vi "TestDCMotors.vi"() -> ()   [LabVIEW 2020]
uses:
  <vilib>/Platform/TimedLoop/XDataNode/timing_clust.ctl
  <vilib>/Platform/TimedLoop/XDataNode/nitl_modes.ctl
  <vilib>/Platform/TimedLoop/XDataNode/wakeup.ctl
  <vilib>/High Genius/HG_WSI_Tookit/Dependencies/Library/CAN/CAN.lvclass
  C:/Program Files (x86)/National Instruments/LabVIEW 2020/vi.lib/High Genius/HG_WSI_Tookit/Dependencies/Library/HG_LIB/HG_LIB.lvclass
  <vilib>/High Genius/HG_WSI_Tookit/Dependencies/Library/Digital Input and Output/Digital Input and Output.lvclass
  <vilib>/High Genius/HG_WSI_Tookit/Dependencies/Library/PWM/PWM.lvclass
  <vilib>/High Genius/HG_WSI_Tookit/Dependencies/Library/TitanENC/TitanENC.lvclass
  <vilib>/Platform/TimedLoop/XDataNode/XDataNode.xnode
  <vilib>/Platform/TimedLoop/XDataNode/XDNodeRunTimeDep.lvlib
  <vilib>/High Genius/HG_WSI_Tookit/Dependencies/Library/HG_LIB/HG_LIB.lvclass
panel:
  in  "s":bool
  in  "error in (no error)":errorcluster
  in  "Servo 1":T1={"Servo 1"=25.6734693877551, "Servo 2"=20.836734693877553, "Servo 3"=0.0} {"Servo 3" min=0.0 max=255.0 step=1.0 scale=10.0..40.0; "Servo 2" min=0.0 max=255.0 step=1.0 scale=10.0..40.0; "Servo 1" min=0.0 max=255.0 step=1.0 scale=10.0..40.0}
  out "Limit L":bool
  out "Limit H":bool
  in  "Motors Renum":cluster{"Num":i32, "Directly":bool, "KM":dbl}[](array[cluster])=[{"Num"=1, "Directly"=TRUE, "KM"=1.0}, {"Num"=3, "Directly"=FALSE, "KM"=1.0}, {"Num"=0, "Directly"=FALSE, "KM"=1.0}, {"Num"=2, "Directly"=TRUE, "KM"=1.0}]
  out "output cluster":T2
  out "Z":dbl
  out "Distance":cluster{"X":dbl, "Y":dbl}
  in  "Reset YAW":bool
  out "YAW (degree)":dbl
  in  "Start":bool
  in  "Drive On":bool
  in  "Drive":dbl[](array[slide])=[0.0, 0.0, -0.01, 1.0] step=1.0 scale=-100.0..100.0
  out "Waveform Chart":i32(graph)
  out "ENC/dt":T3
  out "RPM":T4
  out "ENC True":T5
  out "ENC":T5
  in  "Input":dbl[](array[slide])=[0.0, 0.0, -0.01, 1.0] step=1.0 scale=-100.0..100.0
  in  "Reset Enc":bool
  out "error out":errorcluster
  in  "stop":bool
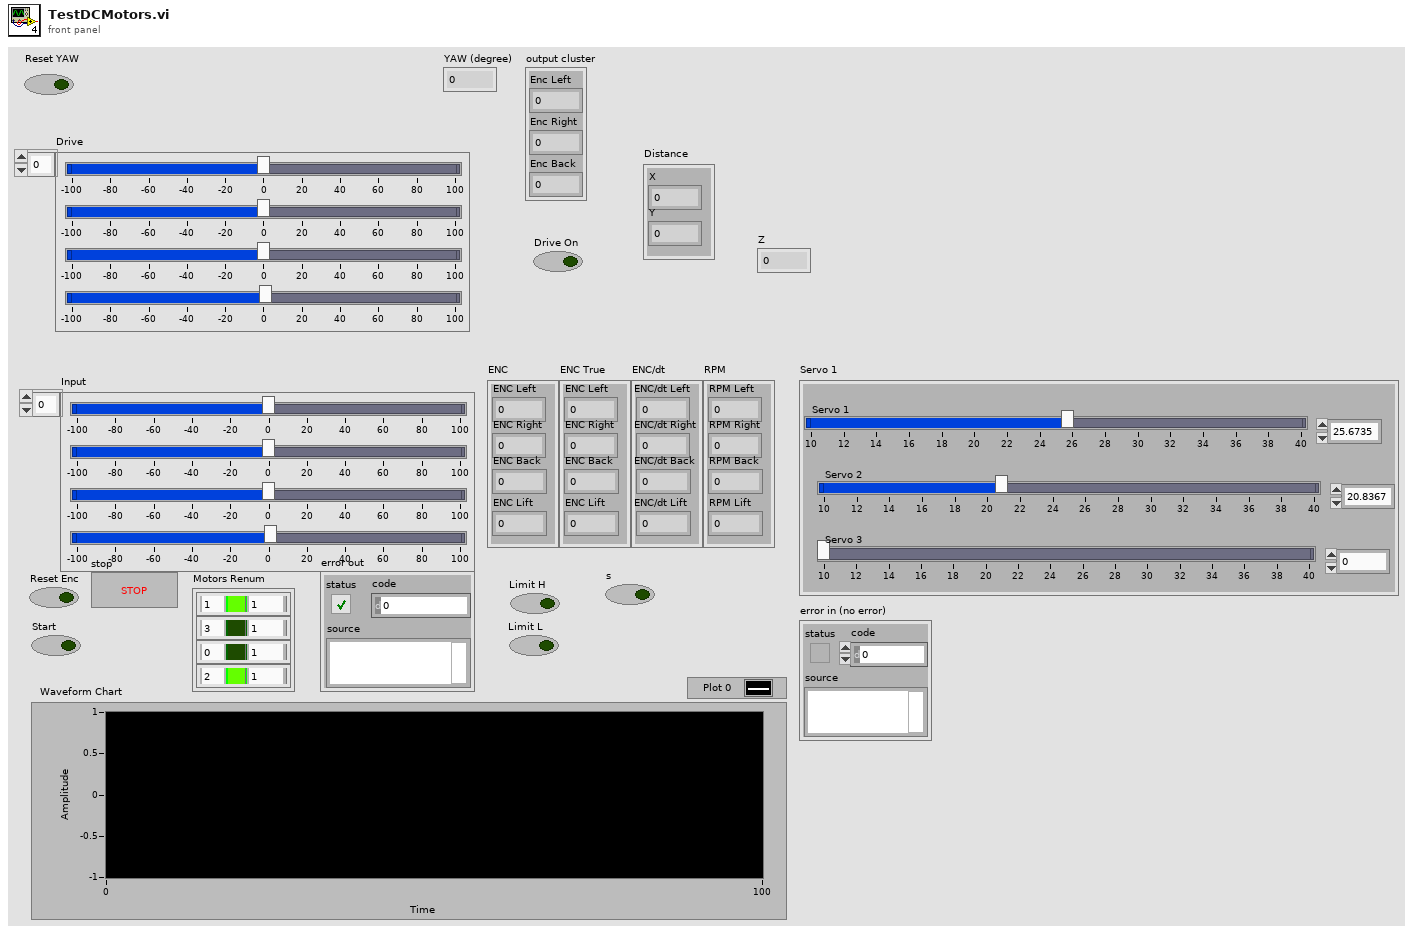
[diagram p1: front panel]
types:
  T1 = cluster{"Servo 1":dbl, "Servo 2":dbl, "Servo 3":dbl}
  T2 = cluster{"Enc Left":dbl, "Enc Right":dbl, "Enc Back":dbl}
  T3 = cluster{"ENC/dt Left":i32, "ENC/dt Right":i32, "ENC/dt Back":i32, "ENC/dt Lift":i32}
  T4 = cluster{"RPM Left":i32, "RPM Right":i32, "RPM Back":i32, "RPM Lift":i32}
  T5 = cluster{"ENC Left":i32, "ENC Right":i32, "ENC Back":i32, "ENC Lift":i32}
  T6 = cluster{"TitanENC 0":refnum<class "TitanENC.lvclass">, "TitanENC 1":refnum<class "TitanENC.lvclass">, "TitanENC 2":refnum<class "TitanENC.lvclass">, "TitanENC 3":refnum<class "TitanENC.lvclass">}
  T7 = cluster{"Limit H":refnum<class "Digital Input and Output.lvclass">, "Limit L":refnum<class "Digital Input and Output.lvclass">}
  T8 = cluster{"Servo 1":refnum<class "PWM.lvclass">, "Servo 2":refnum<class "PWM.lvclass">, "Servo 3":refnum<class "PWM.lvclass">}
  T9 = typedef "XDNodeRunTimeDep.lvlib/timing_clust.ctl" = cluster{"Expected End [f-1]":u64, "Actual End [f-1]":u64, "Finished Late? [f-1]":bool, "Expected End [i-1]":u64, "Actual End [i-1]":u64, "Finished Late? [i-1]":bool, "Expected Start [i]":u64, "Actual Start [i]":u64, "Expected Start [f]":u64, "Actual Start [f]":u64, "Source Name":string, "Structure Name":string, "Period":i64, "Deadline":i64, "Offset":i64, "Start":i64, "Priority":i32, "Timeout":i32, "Mode":T10, "Wakeup Reason":T11, "Error":errorcluster, "Source Type":string, "Secondary Source Type":string, "Global End Time":u64, "Global Start Time":u64, "Frame Duration":u64, "Iteration Duration":u64, "Assigned CPU":i32, "I/O Scan Engine Mode":u32}
  T10 = typedef "XDNodeRunTimeDep.lvlib/nitl_modes.ctl" = enum32{"No Change", "Process missed periods, maintain original phase", "Discard missed periods, maintain original phase", "Process missed periods, ignore original phase", "Discard missed periods, ignore original phase"}
  T11 = typedef "XDNodeRunTimeDep.lvlib/wakeup.ctl" = enum32{"Normal", "Aborted", "Asynchronous wakeup", "Timing source error", "Timed loop error", "Timeout"}
  T12 = cluster{"Limit H out":refnum<class "Digital Input and Output.lvclass">, "Limit L out":refnum<class "Digital Input and Output.lvclass">}
  T13 = cluster{"Servo 1 out":refnum<class "PWM.lvclass">, "Servo 2 out":refnum<class "PWM.lvclass">, "Servo 3 out":refnum<class "PWM.lvclass">}
  T14 = cluster{"TitanENC out":refnum<class "TitanENC.lvclass">, "TitanENC out":refnum<class "TitanENC.lvclass">, "TitanENC out":refnum<class "TitanENC.lvclass">, "TitanENC out":refnum<class "TitanENC.lvclass">}
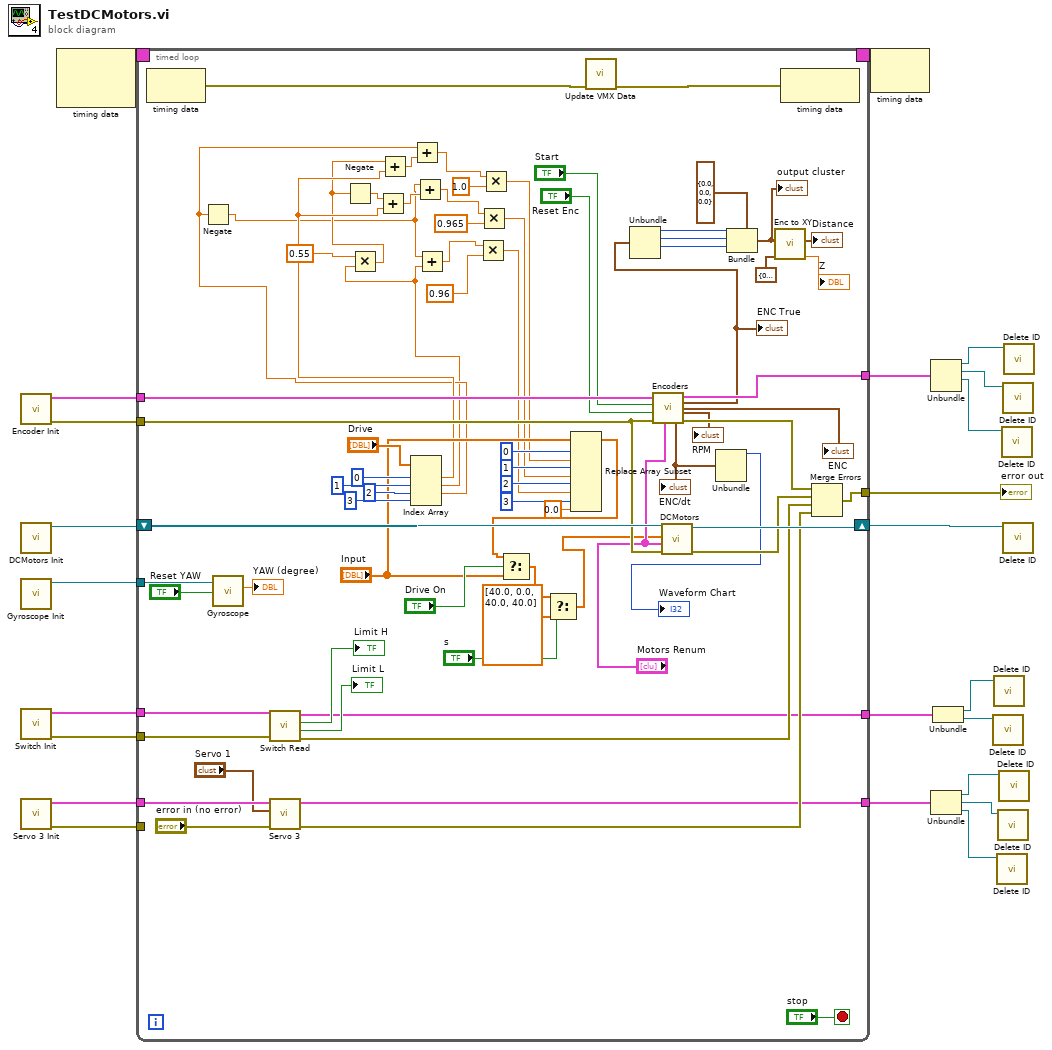
[diagram p0: block diagram]
diagram:
  n1 = call "Encoder Init.vi"() -> ("error out"=w14:errorcluster, "TitanENC out"=w15:T6)  [unwired: 10 in]
  n2 = call "DCMotors Init.vi"() -> ("DC Motors"=w13:refnum<class "CAN.lvclass">)  [unwired: 10 in, 1 out]
  n3 = call "Gyroscope Init.vi"() -> ("Gyroscope"=w12:refnum<class "IMU.lvclass">)  [unwired: 10 in, 1 out]
  n4 = call "Switch Init.vi"() -> ("error out"=w10:errorcluster, "Switch"=w11:T7)  [unwired: 10 in]
  n5 = call "Servo 3 Init.vi"() -> ("error out"=w8:errorcluster, "Servo"=w9:T8)  [unwired: 10 in]
  n6 = node-c288() -> (w23:T9)  [unwired: 2 in]
  n7 = timed-loop {
    timing: w23 -> [_]
    timing-out: [_] -> w22
    shift-right: [w98] -> w21
    shift-left: w13 -> [w99]
    tunnel: w14 -> [w93]
    tunnel: w15 -> [w94]
    tunnel: [w91] -> w20
    tunnel: [w88] -> w17
    tunnel: w12 -> [w52]
    tunnel: w11 -> [w39]
    tunnel: w10 -> [w38]
    tunnel: w9 -> [w35]
    tunnel: w8 -> [_]
    tunnel: [w31] -> w7
    tunnel: [w30] -> w3
    stop <- "stop" stop-if-true
    n8 = node-c288() -> (w97:errorcluster)  [unwired: 1 in]
    n9 = call "Gyroscope.vi"("Reset YAW"="Reset YAW", "IMU in"=w52) -> ("YAW (degree)"=→"YAW (degree)":dbl)  [unwired: 5 in, 4 out]
    n10 = call "Switch Read.vi"("error in (no error)"=w38, "HG_LIB in"=w39) -> ("error out"=w33:errorcluster, "Limit L"=→"Limit L":bool, "Limit H"=→"Limit H":bool, "HG_LIB out"=w30:T12)  [unwired: 6 in]
    n11 = call "Servo 3.vi"("error in (no error)"="error in (no error)", "Servo"="Servo 1", "PWM in"=w35) -> ("error out"=w34:errorcluster, "PWM out"=w31:T13)  [unwired: 7 in]
    n12 = Index Array(array="Drive", index #1=0 ("index"), index #2=1 ("index"), index #3=2 ("index"), index #4=3 ("index")) -> (element #1=w67:dbl, element #2=w54:dbl, element #3=w58:dbl)  [unwired: 1 out]
    n13 = Negate(x=w58) -> (-x=w53:dbl)
    n14 = Multiply(x=0.55, y=w54) -> (x*y=w61:dbl)
    n15 = Negate(x=w61) -> (-x=w62:dbl)
    n16 = Add(x=w62, y=w67) -> (x+y=w57:dbl)
    n17 = Add(x=w61, y=w67) -> (x+y=w60:dbl)
    n18 = Add(x=w58, y=w60) -> (x+y=w59:dbl)
    n19 = Add(x=w53, y=w57) -> (x+y=w56:dbl)
    n20 = Add(x=w53, y=w54) -> (x+y=w55:dbl)
    n21 = Multiply(x=w55, y=0.96) -> (x*y=w64:dbl)
    n22 = Multiply(x=w56, y=0.965) -> (x*y=w68:dbl)
    n23 = Multiply(x=w59, y=1.0) -> (x*y=w69:dbl)
    n24 = Replace Array Subset(array="Input", new element #1=w69, index #1=0 ("index"), new element #2=w68, index #2=1 ("index"), new element #3=w64, index #3=2 ("index"), new element #4=0.0 ("new element/subarray"), index #4=3 ("index")) -> (w78:dbl[])
    n25 = Select(t=w78, s="Drive On", f="Input") -> (s? t:f=w27:dbl[])
    n26 = Select(t=dbl[] [40.0, 0.0, 40.0, 40.0], s="s", f=w27) -> (s? t:f=w25:dbl[])
    n27 = call <vilib>:"Update VMX Data.vi"("error in (no error)"=w97) -> ("error out"=w96:errorcluster)  [unwired: 10 in]
    n28 = call "Encoders.vi"("Motors Renum"="Motors Renum", "error in (no error)"=w93, "Reset Enc"="Reset Enc", "Start"="Start", "TitanENC in"=w94) -> ("error out"=w90:errorcluster, "RPM"=→"RPM":T4, "ENC True"=w49:T5, "TitanENC out"=w91:T14, "ENC/dt"=w86:T3, "ENC"=→"ENC":T5)  [unwired: 1 in]
    "ENC True" <- w49
    "ENC/dt" <- w86
    n29 = Unbundle(w49) -> ("ENC Left"=w47:i32, "ENC Right"=w46:i32, "ENC Back"=w45:i32)  [unwired: 1 out]
    n30 = call "DCMotors.vi"("error in"=w93, "Motors Renum"="Motors Renum", "Input"=w25, "CAN in"=w99) -> ("error out"=w89:errorcluster, "CAN out"=w98:refnum<class "CAN.lvclass">)  [unwired: 6 in]
    n31 = Unbundle(w86) -> ("ENC/dt Left"=→"Waveform Chart":i32)  [unwired: 3 out]
    n32 = Bundle(cluster=T2 {"Enc Left"=0.0, "Enc Right"=0.0, "Enc Back"=0.0} ("Encoders"), "Enc Left"=w47, "Enc Right"=w46, "Enc Back"=w45) -> (w44:T2)
    "output cluster" <- w44
    n33 = call "Enc to XY.vi"("Factor"=cluster{"Kx":dbl, "Ky":dbl, "Kz":dbl} {"Kx"=0.02114, "Ky"=0.0245, "Kz"=0.0705}, "Encoders"=w44) -> ("Z"=→"Z":dbl, "Distance"=→"Distance":cluster{"X":dbl, "Y":dbl})  [unwired: 8 in]
    n34 = node-c288(w96) -> ()  [unwired: 1 out]
    n35 = Merge Errors(w90, w89, w33, w34) -> (w88:errorcluster)
  }
  "error out" <- w17
  n36 = node-c288(w22) -> ()  [unwired: 1 out]
  n37 = Unbundle(w20) -> ("TitanENC out"=w19:refnum<class "TitanENC.lvclass">, "TitanENC out"=w16:refnum<class "TitanENC.lvclass">, "TitanENC out"=w18:refnum<class "TitanENC.lvclass">)  [unwired: 1 out]
  n38 = Unbundle(w7) -> ("Servo 1 out"=w6:refnum<class "PWM.lvclass">, "Servo 2 out"=w5:refnum<class "PWM.lvclass">, "Servo 3 out"=w4:refnum<class "PWM.lvclass">)
  n39 = Unbundle(w3) -> ("Limit H out"=w1:refnum<class "Digital Input and Output.lvclass">, "Limit L out"=w2:refnum<class "Digital Input and Output.lvclass">)
  n40 = call <vilib>:"Delete ID.vi"("HG_LIB in"=w2) -> ()  [unwired: 9 in, 2 out]
  n41 = call <vilib>:"Delete ID.vi"("HG_LIB in"=w1) -> ()  [unwired: 9 in, 2 out]
  n42 = call <vilib>:"Delete ID.vi"("HG_LIB in"=w4) -> ()  [unwired: 9 in, 2 out]
  n43 = call <vilib>:"Delete ID.vi"("HG_LIB in"=w5) -> ()  [unwired: 9 in, 2 out]
  n44 = call <vilib>:"Delete ID.vi"("HG_LIB in"=w6) -> ()  [unwired: 9 in, 2 out]
  n45 = call <vilib>:"Delete ID.vi"("HG_LIB in"=w18) -> ()  [unwired: 9 in, 2 out]
  n46 = call <vilib>:"Delete ID.vi"("HG_LIB in"=w16) -> ()  [unwired: 9 in, 2 out]
  n47 = call <vilib>:"Delete ID.vi"("HG_LIB in"=w21) -> ()  [unwired: 9 in, 2 out]
  n48 = call <vilib>:"Delete ID.vi"("HG_LIB in"=w19) -> ()  [unwired: 9 in, 2 out]
